vi "Execute.vi"(0 "Session Handle in":T1, 11 "error in (no error)":errorcluster) -> (4 "Session Handle out":T1, 15 "error out":errorcluster)   [LabVIEW 2020, in "HTS.lvlib" / "Execution.lvclass"]
uses:
  Execution.lvclass
  Typedefs/Session Handle.ctl
  Execution.lvclass/Execution.ctl
  VariableContainer/Get Ref Prop.vi
  SequenceFile/Get Ref Prop.vi
  Engine/Get Engine Ref.vi
  SequenceFile/SequenceFile.lvclass
  Engine/Engine.lvclass
  VariableContainer/VariableContainer.lvclass
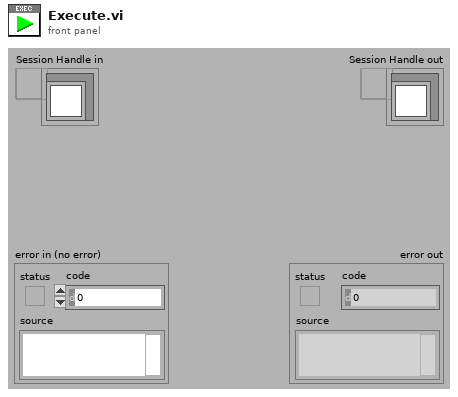
[diagram p1: front panel]
types:
  T1 = typedef "HTS.lvlib/Execution.lvclass/Session Handle.ctl" = refnum<data-value>
  T2 = typedef "HTS.lvlib/Engine.lvclass/Session Handle.ctl" = refnum<data-value>
  T3 = typedef "HTS.lvlib/SequenceFile.lvclass/Session Handle.ctl" = refnum<data-value>
  T4 = typedef "HTS.lvlib/VariableContainer.lvclass/Session Handle.ctl" = refnum<data-value>
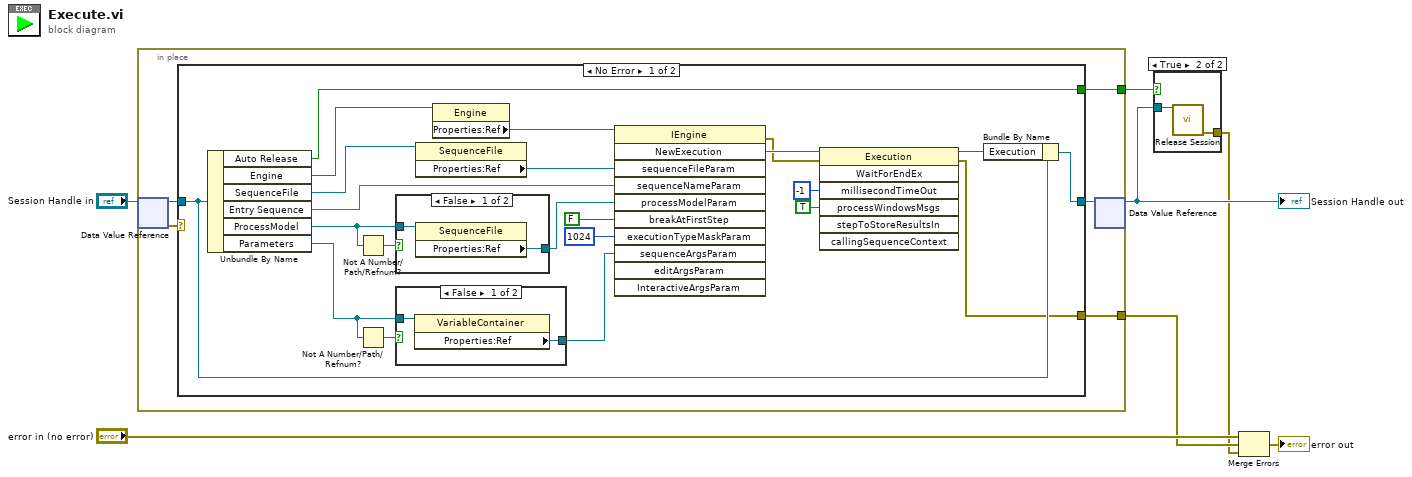
[diagram p0: block diagram]
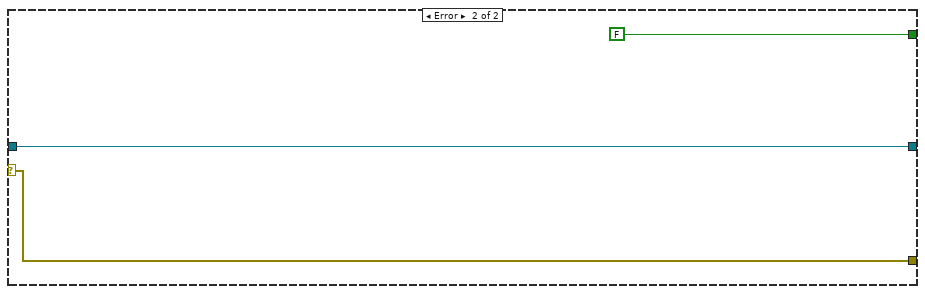
[diagram p4: hidden frame]
diagram:
  n1 = in-place {
    in-place-border: [w10] -> w4
    in-place-border: [w8] -> w2
    n2 = in-place-dvr #1("Session Handle in") -> (w12:refnum<class "Execution.lvclass">, w9:errorcluster)
    n3 = case shown="No Error" w9 {
      selector: w9 -> [_ w41]
      tunnel: w12 -> [w22 w40]
      tunnel: [w21 w40] -> w11
      tunnel: [w20 FALSE ("Auto Release")] -> w10
      tunnel: [w13 w41] -> w8
      frame No Error {
        n4 = Unbundle By Name(w22) -> ("Auto Release"=w20:bool, "Engine"=w34:T2, "SequenceFile"=w32:T3, "Entry Sequence"=w30:string, "ProcessModel"=w27:T3, "Parameters"=w24:T4)
        n5 = Not A Number/Path/Refnum?(number/path/refnum=w27) -> (NaN/Path/Refnum?=w28:bool)
        n6 = Not A Number/Path/Refnum?(number/path/refnum=w24) -> (NaN/Path/Refnum?=w25:bool)
        n7 = case shown="False" w28 {
          tunnel: w27 -> [w38 _]
          tunnel: [w37 _] -> w26
          frame False {
            n8 = property class="SequenceFile"(reference=w38) -> ("Properties:Ref"=w37:refnum<k7>)  [unwired: 1 in, 2 out]
          }
          frame True {
          }
        }
        n9 = case shown="False" w25 {
          tunnel: w24 -> [w36 _]
          tunnel: [w35 _] -> w23
          frame False {
            n10 = property class="VariableContainer"(reference=w36) -> ("Properties:Ref"=w35:refnum<k7>)  [unwired: 1 in, 2 out]
          }
          frame True {
          }
        }
        n11 = property class="SequenceFile"(reference=w32) -> ("Properties:Ref"=w31:refnum<k7>)  [unwired: 1 in, 2 out]
        n12 = property class="Engine"(reference=w34) -> ("Properties:Ref"=w33:refnum<k7>)  [unwired: 1 in, 2 out]
        n13 = invoke class="IEngine" method="NewExecution"(reference=w33, "sequenceFileParam"=w31, "sequenceNameParam"=w30, "processModelParam"=w26, "breakAtFirstStep"=FALSE, "executionTypeMaskParam"=1024, "sequenceArgsParam"=w23) -> (error out=w14:errorcluster, "NewExecution"=w18:refnum<k7>)  [unwired: 4 in, 9 out]
        n14 = invoke class="Execution" method="WaitForEndEx"(reference=w18, error in=w14, "millisecondTimeOut"=-1, "processWindowsMsgs"=TRUE) -> (reference out=w17:refnum<k7>, error out=w13:errorcluster)  [unwired: 3 in, 5 out]
        n15 = Bundle By Name(cluster=w22, "Execution"=w17) -> (w21:refnum<class "Execution.lvclass">)
      }
      frame Error {
      }
    }
    n16 = in-place-dvr #1(w11) -> (w5:T1)  [unwired: 1 out]
  }
  "Session Handle out" <- w5
  n17 = case shown="True" w4 {
    tunnel: w5 -> [_ w43]
    tunnel: [_ w42] -> w1
    frame False {
    }
    frame True {
      n18 = call "Release Session.vi"("Session Handle"=w43) -> ("error out"=w42:errorcluster)  [unwired: 14 in]
    }
  }
  n19 = Merge Errors("error in (no error)", w2, w1) -> (→"error out":errorcluster)
